vi "Catapult Loop.vi"   [LabVIEW 2015]
uses:
  Robot Global Data.vi
  <vilib>/Rock Robotics/WPI/Solenoid/Deprecated/WPI_SolenoidSetBool.vi
types:
  T1 = typedef "Catapult Command Cluster.ctl" = cluster{"Command":T2, "Mode":T3, "Override Trigger Sensor":bool, "High Power Shot?":bool, "Vision?":bool}
  T2 = typedef "Shooter Commands.ctl" = enum16{"Idle", "Prime Shooter", "Shoot"}
  T3 = typedef "Shoot Modes Enum.ctl" = enum16{"Manual", "Safe", "Auto"}
  T4 = typedef "WPI_SwitchDevRef.ctl" = cluster{"DevStatus":errorcluster, "DIO Channel":T5, "CntIndex":T6, "Normally Closed":bool}
  T5 = typedef "FPGA_DIOChannel.ctl" = enum8{"DIO 0", "DIO 1", "DIO 2", "DIO 3", "DIO 4", "DIO 5", "DIO 6", "DIO 7", "DIO 8", "DIO 9", "DIO MXP 0", "DIO MXP 1", "DIO MXP 2", "DIO MXP 3", "DIO MXP 4", "DIO MXP 5", "DIO MXP 6", "DIO MXP 7", "DIO MXP 8", "DIO MXP 9", "DIO MXP 10", "DIO MXP 11", "DIO MXP 12", "DIO MXP 13", "DIO MXP 14", "DIO MXP 15", "Invalid"}
  T6 = typedef "FPGA_CounterCtrSystemIndex.ctl" = enum8{"Ctr 0", "Ctr 1", "Ctr 2", "Ctr 3", "Ctr 4", "Ctr 5", "Ctr 6", "Ctr 7", "Invalid"}
  T7 = typedef "WPI_DigitalInputDevRef.ctl" = cluster{"DevStatus":errorcluster, "DIO Channel":T5}
  T8 = typedef "WPI_SolenoidDevRef.ctl" = cluster{"DevStatus":errorcluster, "Pneumatics Control Module":u8, "Forward Solenoid Channel":T9, "Reverse Solenoid Channel":T9}
  T9 = typedef "WPI_SolenoidChannel.ctl" = enum8{"Solenoid 0", "Solenoid 1", "Solenoid 2", "Solenoid 3", "Solenoid 4", "Solenoid 5", "Solenoid 6", "Solenoid 7", "Invalid"}
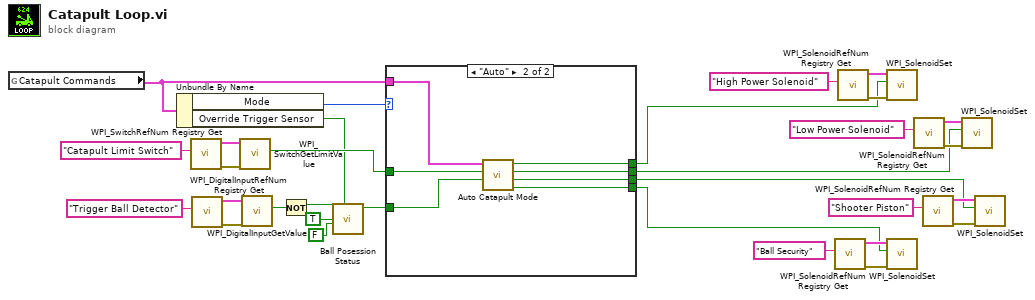
[diagram p0: block diagram]
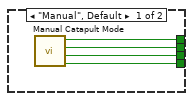
[diagram p2: hidden frame]
diagram:
  n1 = global read "Robot Global Data.vi" "Catapult Commands"() -> (w2:T1)
  n2 = Unbundle By Name(w2) -> ("Mode"=w3:T3, "Override Trigger Sensor"=w1:bool)
  n3 = call <vilib>:"WPI_SwitchRefNum Registry Get.vi"("refnum name"="Catapult Limit Switch") -> ("error out"=w30:errorcluster, "SwitchDevRef"=w29:T4)  [unwired: 9 in]
  n4 = call <vilib>:"WPI_DigitalInputRefNum Registry Get.vi"("refnum name"="Trigger Ball Detector") -> ("error out"=w10:errorcluster, "DigitalInputDevRef"=w9:T7)  [unwired: 9 in]
  n5 = call <vilib>:"WPI_SwitchGetLimitValue.vi"("error in (no error)"=w30, "SwitchDevRef"=w29) -> ("Switch Pressed"=w28:bool)  [unwired: 7 in, 2 out]
  n6 = call <vilib>:"WPI_DigitalInputGetValue.vi"("error in (no error)"=w10, "DigitalInputDevRef"=w9) -> ("Value"=w6:bool)  [unwired: 7 in, 2 out]
  n7 = Not(x=w6) -> (.not. x?=w5:bool)
  n8 = call "Ball Posession Status.vi"("Override?"=w1, "Logical Exit?"=FALSE, "Using Sensor?"=TRUE, "Sensor"=w5) -> ("Ball Posessed?"=w4:bool)  [unwired: 7 in]
  n9 = case shown="\"Auto\"" w3 {
    tunnel: w28 -> [_ w42]
    tunnel: [w35 w41] -> w16
    tunnel: [w34 w40] -> w19
    tunnel: [w33 w39] -> w22
    tunnel: [w32 w38] -> w12
    tunnel: w4 -> [_ w37]
    tunnel: w2 -> [_ w36]
    frame "Manual", Default {
      n10 = call "Manual Catapult Mode.vi"() -> ("Claw?"=w32:bool, "Pin Shooter?"=w33:bool, "Low Power Solenoid"=w34:bool, "High Power Solenoid"=w35:bool)  [unwired: 8 in]
    }
    frame "Auto" {
      n11 = call "Auto Catapult Mode.vi"("Ball Loaded?"=w37, "Limit Switch Activated?"=w42, "Catapult Commands"=w36) -> ("Secure Ball?"=w38:bool, "Pinned?"=w39:bool, "Low Power Solenoid"=w40:bool, "High Power Solenoid"=w41:bool)  [unwired: 5 in]
    }
  }
  n12 = call <vilib>:"WPI_SolenoidRefNum Registry Get.vi"("refnum name"="Ball Security") -> ("error out"=w14:errorcluster, "SolenoidDevRef"=w15:T8)  [unwired: 9 in]
  n13 = call <vilib>:"WPI_SolenoidRefNum Registry Get.vi"("refnum name"="High Power Solenoid") -> ("error out"=w18:errorcluster, "SolenoidDevRef"=w17:T8)  [unwired: 9 in]
  n14 = call-poly <vilib>:"WPI_SolenoidSet.vi"("error in (no error)"=w18, "Value"=w16, "SolenoidDevRef"=w17) -> ()  [unwired: 7 in, 2 out]
  n15 = call-poly <vilib>:"WPI_SolenoidSet.vi"("error in (no error)"=w14, "Value"=w12, "SolenoidDevRef"=w15) -> ()  [unwired: 7 in, 2 out]
  n16 = call <vilib>:"WPI_SolenoidRefNum Registry Get.vi"("refnum name"="Low Power Solenoid") -> ("error out"=w21:errorcluster, "SolenoidDevRef"=w20:T8)  [unwired: 9 in]
  n17 = call <vilib>:"WPI_SolenoidRefNum Registry Get.vi"("refnum name"="Shooter Piston") -> ("error out"=w24:errorcluster, "SolenoidDevRef"=w23:T8)  [unwired: 9 in]
  n18 = call-poly <vilib>:"WPI_SolenoidSet.vi"("error in (no error)"=w21, "Value"=w19, "SolenoidDevRef"=w20) -> ()  [unwired: 7 in, 2 out]
  n19 = call-poly <vilib>:"WPI_SolenoidSet.vi"("error in (no error)"=w24, "Value"=w22, "SolenoidDevRef"=w23) -> ()  [unwired: 7 in, 2 out]
